vi "多列列表框上色.vi"(4 "颜色":cluster{"偶数行颜色盒":u32, "奇数行颜色盒":u32}={"偶数行颜色盒"=16763272, "奇数行颜色盒"=12439011}, 6 "同色行数":i32, 8 "错误输入（无错误）":errorcluster, 9 "行列总数":cluster{"列总数":i32, "行总数":i32}, 10 "起始行列":cluster{"行":i32, "列":i32}, 11 "多列列表框 2":refnum<vi>) -> (0 "错误输出":errorcluster, 3 "多列列表框":refnum<vi>)   [LabVIEW 2014, in "表格.lvlib" / "表格上色.lvlib"]
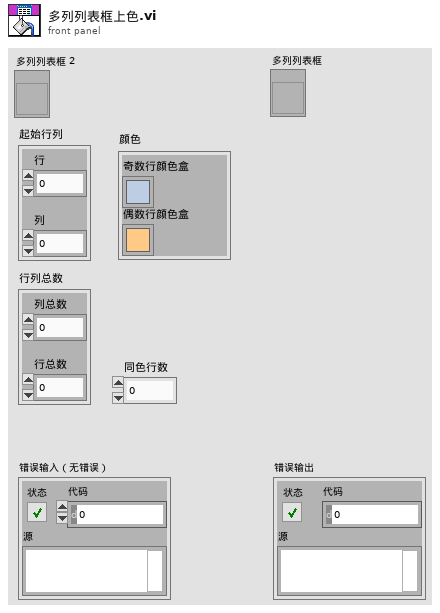
[diagram p1: front panel]
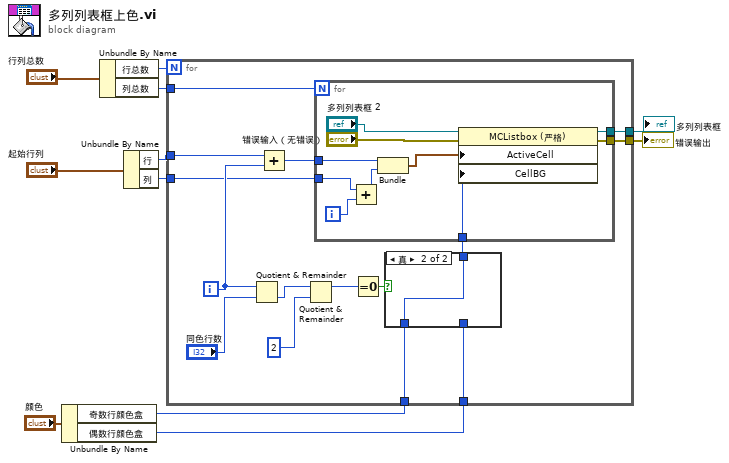
[diagram p0: block diagram]
diagram:
  n1 = Unbundle By Name("颜色") -> ("奇数行颜色盒"=w7:u32, "偶数行颜色盒"=w6:u32)
  n2 = Unbundle By Name("行列总数") -> ("行总数"=w10:i32, "列总数"=w9:i32)
  n3 = Unbundle By Name("起始行列") -> ("行"=w4:i32, "列"=w3:i32)
  n4 = for {
    N: w10 -> [_]
    tunnel: w9 -> [w20]
    tunnel: w7 -> [w19]
    tunnel: w6 -> [w18]
    tunnel: w4 -> [w16]
    tunnel: w3 -> [w14]
    tunnel: [w13] -> w2
    tunnel: [w12] -> w1
    i -> [w17]
    n5 = Quotient & Remainder(x=w17, y="同色行数") -> (floor(x/y)=w23:i32)  [unwired: 1 out]
    n6 = Add(x=w16, y=w17) -> (x+y=w15:i32)
    n7 = Quotient & Remainder(x=w23, y=2) -> (x-y*floor(x/y)=w21:i32)  [unwired: 1 out]
    n8 = Equal To 0?(x=w21) -> (x = 0?=w26:bool)
    n9 = case shown="真" w26 {
      tunnel: [w27 w28] -> w25
      tunnel: w19 -> [_ w28]
      tunnel: w18 -> [w27 _]
      frame False {
      }
      frame True {
      }
    }
    n10 = for {
      N: w20 -> [_]
      tunnel: w15 -> [w38]
      tunnel: w25 -> [w36]
      tunnel: w14 -> [w34]
      tunnel: [w30] -> w13
      tunnel: [w29] -> w12
      i -> [w35]
      n11 = Add(x=w34, y=w35) -> (x+y=w33:i32)
      n12 = Bundle(w38, w33) -> (w37:cluster{i32, i32})  [unwired: 1 in]
      n13 = property on="属性节点" class="MCListbox (严格)"(reference="多列列表框 2", error in="错误输入（无错误）", "ActiveCell"=w37, "CellBG"=w36) -> (reference out=w29:refnum<vi>, error out=w30:errorcluster)
    }
  }
  "错误输出" <- w2
  "多列列表框" <- w1
